vi "scanSubDir.vi"(1 "path":path) -> (0 "Array":path[](array[path]))   [LabVIEW 2009]
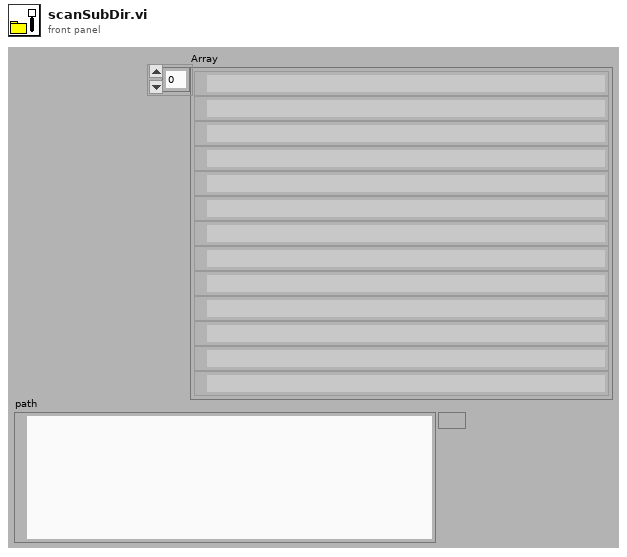
[diagram p1: front panel]
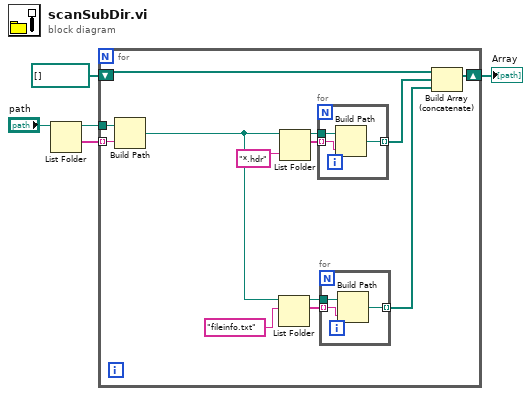
[diagram p0: block diagram]
diagram:
  n1 = List Folder(path="path") -> (path out=w3:path, folder names=w4:string[])  [unwired: 3 in, 2 out]
  n2 = for {
    tunnel: w4 -> [w18] mode=indexing
    tunnel: w3 -> [w17]
    shift-right: [w13] -> w1
    shift-left: path[] [] -> [w11]
    n3 = Build Path(base path=w17, name or relative path=w18) -> (appended path=w10:path)
    n4 = List Folder(path=w10, pattern="fileinfo.txt") -> (path out=w8:path, filenames=w7:string[])  [unwired: 2 in, 2 out]
    n5 = List Folder(path=w10, pattern="*.hdr") -> (path out=w15:path, filenames=w14:string[])  [unwired: 2 in, 2 out]
    n6 = for {
      tunnel: w15 -> [w24]
      tunnel: w14 -> [w23] mode=indexing
      tunnel: [w22] -> w12 mode=indexing
      n7 = Build Path(base path=w24, name or relative path=w23) -> (appended path=w22:path)
    }
    n8 = for {
      tunnel: w8 -> [w21]
      tunnel: w7 -> [w20] mode=indexing
      tunnel: [w19] -> w6 mode=indexing
      n9 = Build Path(base path=w21, name or relative path=w20) -> (appended path=w19:path)
    }
    n10 = Build Array (concatenate)(w11, w12, w6) -> (w13:path[])
  }
  "Array" <- w1
